vi "Pump_commands_Testcode.vi"() -> ()   [LabVIEW 2024]
uses:
  <vilib>/Instr/_visa.llb/VISA Find Search Mode.ctl
  ee3f6e9a-4254-40fb-8a6d-f40dbbb11eb6.vi
  <vilib>/regexp/Match Regular Expression.xnode
panel:
  out "element 2":u8
  out "element":u8
  out "read buffer":string
  out "Error":string
  out "Error present":bool
  out "Ready":bool
  out "Boolean array":bool[](array[boolean])
  out "Numeric 2":u8
  out "unsigned byte array":u8[](array[numeric])
  in  "Send":bool
  out "appended array":T1(array[ring])
  out "Responce array":string[](array[string])
  out "error out 2":errorcluster
  out "Numeric":i32
  out "Pump found":bool
  out "String":string
  in  "stop":bool
  in  "Enum":T2(ring)
  out "Array":string[](array[string])
  # "Hvis pumpen køre hurtigere end 17 laver den cavitations eller får væsken til at kåge"
  # "5"
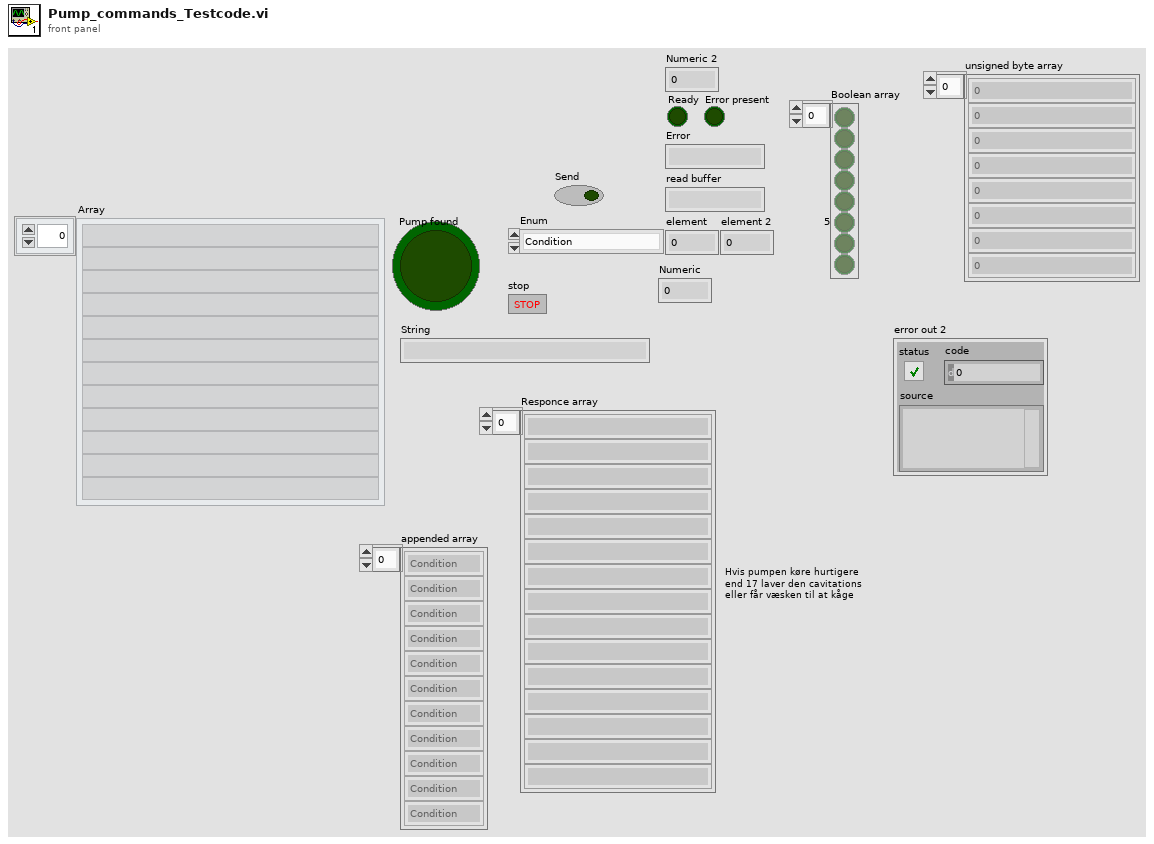
[diagram p1: front panel]
types:
  T1 = enum16{"Condition", "Pump out", "Pump in", "Initiate"}[]
  T2 = enum16{"Condition", "Pump out", "Pump in", "Initiate"}
  T3 = typedef "VISA Find Search Mode.ctl" = u32
  T4 = cluster{"VISA resource name":refnum<visa-resource-name>, "error out":errorcluster}
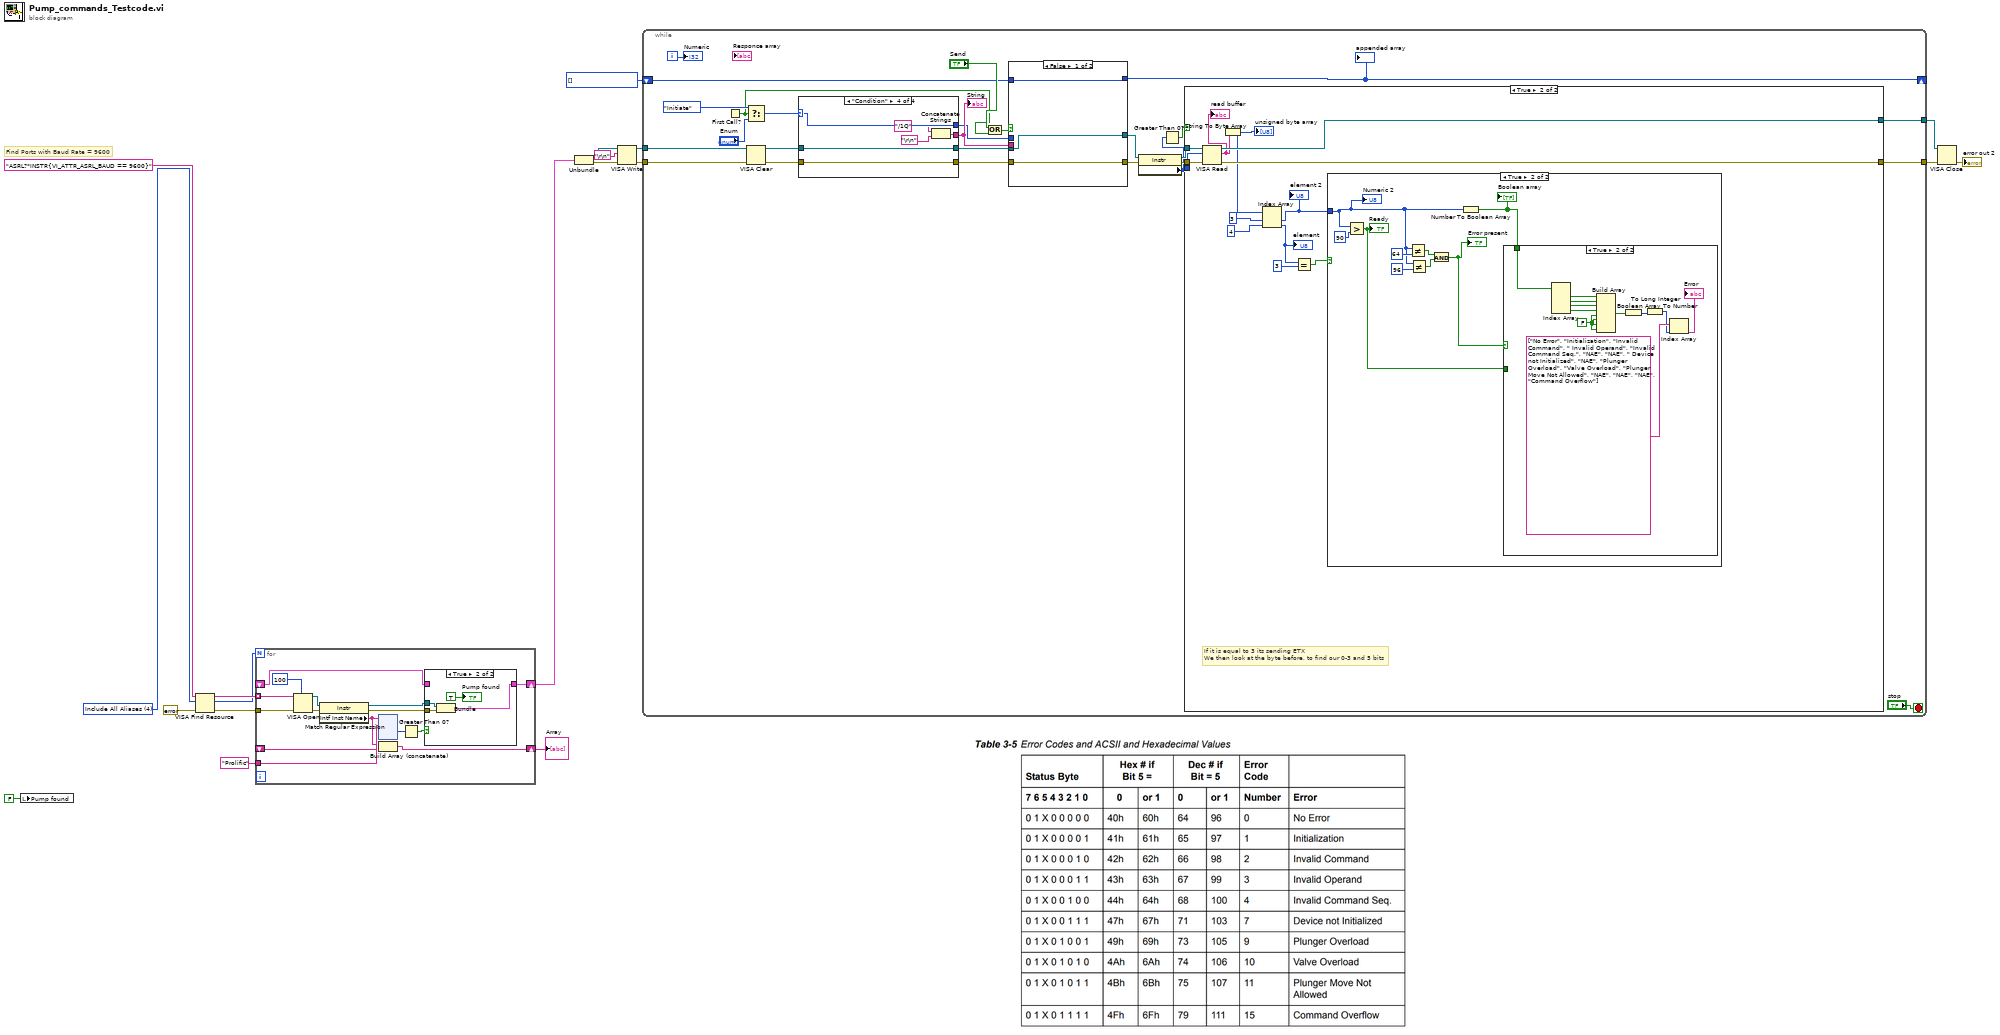
[diagram p0: block diagram]
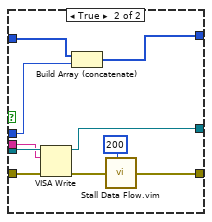
[diagram p5: hidden frame]
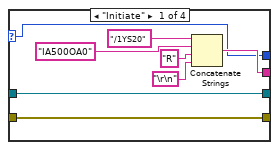
[diagram p6: hidden frame]
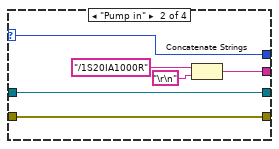
[diagram p7: hidden frame]
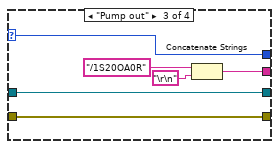
[diagram p8: hidden frame]
diagram:
  w1 = T1 [] items=["Condition", "Pump out", "Pump in", "Initiate"]
  w16 = T3 4 items=["Canonical Names Only"=0, "Aliases Only"=2, "Include Matching Aliases"=3, "Include All Aliases"=4] ("Search Mode")
  # "Find Ports with Baud Rate = 9600"
  n1 = local write "Pump found"(FALSE ("Pump found")) -> ()
  n2 = VISA Find Resource(8:errorcluster {"status"=FALSE, "code"=0, "source"=""} ("error in"), 10:w16, 11:"ASRL?*INSTR{VI_ATTR_ASRL_BAUD == 9600}" ("expression (\"?*\")")) -> (0:w18:errorcluster, 2:w11:u32, 3:w19:string[])
  n3 = for {
    N: w11 -> [_]
    tunnel: w19 -> [w34] mode=indexing
    tunnel: w18 -> [w31]
    shift-right: [w30] -> w14
    shift-left: _ -> [w29]
    tunnel: "Prolific" -> [w24]
    shift-right: [w21] -> w10
    shift-left: _ -> [w20]
    n4 = VISA Open(timeout (0)=u32 100 ("VISA Open timeout (0)"), error in (no error)=w31, VISA resource name=w34) -> (VISA resource name=w33:refnum<visa-resource-name>, error out=w32:errorcluster)  [unwired: 2 in]
    n5 = property class="Instr"(reference=w33, error in=w32) -> (reference out=w26:refnum<visa-resource-name>, error out=w25:errorcluster, "Intf Inst Name"=w22:string)
    n6 = xnode "Match Regular Expression"("input string"=w22, "regular expression"=w24) -> ("offset past match"=w28:i32)  [unwired: 4 in, 4 out]
    n7 = Build Array (concatenate)(w22, w20) -> (w21:string[])
    n8 = Greater Than 0?(x=w28) -> (x > 0?=w27:bool)
    n9 = case shown="True" w27 {
      tunnel: w26 -> [_ w156]
      tunnel: w25 -> [_ w155]
      tunnel: [w152 w154] -> w30
      tunnel: w29 -> [w152 _]
      frame False {
      }
      frame True {
        n10 = Bundle("VISA resource name"=w156, "error out"=w155) -> (w154:T4)  [unwired: 1 in]
        "Pump found" <- TRUE
      }
    }
  }
  "Array" <- w10
  n11 = Unbundle(w14) -> ("VISA resource name"=w8:refnum<visa-resource-name>, "error out"=w9:errorcluster)
  n12 = VISA Write(VISA resource name=w8, write buffer="\r\n", error in (no error)=w9) -> (VISA resource name out=w2:refnum<visa-resource-name>, error out=w3:errorcluster)  [unwired: 1 out]
  n13 = while {
    tunnel: [w177] -> w6
    tunnel: [w178] -> w5
    tunnel: w3 -> [w175]
    tunnel: w2 -> [w174]
    shift-right: [w159] -> _
    shift-left: w1 -> [w160]
    i -> [w181]
    stop <- "stop" stop-if-true
    n14 = First Call?() -> (First Call?: T/F=w163:bool)
    n15 = Select(t=T2."Initiate", s=w163, f="Enum") -> (s? t:f=w165:T2)
    n16 = VISA Clear(VISA resource name=w174, error in (no error)=w175) -> (VISA resource name out=w172:refnum<visa-resource-name>, error out=w173:errorcluster)
    n17 = case shown="\"Condition\"" w165 {
      selector: w165 -> [w231 w239 w245 w254]
      tunnel: [w238 w244 w250 w256] -> w170
      tunnel: w172 -> [w238 w244 w250 w256]
      tunnel: [w237 w243 w249 w255] -> w171
      tunnel: w173 -> [w237 w243 w249 w255]
      tunnel: [w233 w241 w246 w253] -> w168
      tunnel: [w231 w239 w245 w254] -> w161
      frame "Initiate" {
        n18 = Concatenate Strings("/1YS20", "IA500OA0" ("string"), "R" ("string"), "\r\n") -> (w233:string)
      }
      frame "Pump in" {
        n19 = Concatenate Strings("/1S20IA1000R", "\r\n") -> (w241:string)
      }
      frame "Pump out" {
        n20 = Concatenate Strings("/1S20OA0R", "\r\n") -> (w246:string)
      }
      frame "Condition" {
        n21 = Concatenate Strings("/1Q", "\r\n") -> (w253:string)
      }
    }
    "String" <- w168
    n22 = Or(x="Send", y=w163) -> (x .or. y?=w162:bool)
    n23 = case shown="False" w162 {
      tunnel: [w219 w222] -> w176
      tunnel: w171 -> [w219 w230]
      tunnel: w170 -> [w220 w229]
      tunnel: [w220 w228] -> w169
      tunnel: w168 -> [_ w227]
      tunnel: w161 -> [_ w224]
      tunnel: w160 -> [w218 w226]
      tunnel: [w218 w225] -> w159
      frame False {
      }
      frame True {
        n24 = VISA Write(VISA resource name=w229, write buffer=w227, error in (no error)=w230) -> (VISA resource name out=w228:refnum<visa-resource-name>, error out=w223:errorcluster)  [unwired: 1 out]
        n25 = Build Array (concatenate)(w226, w224) -> (w225:T1)
        n26 = call "Stall Data Flow.vim"("value in"=w223, "milliseconds to wait"=u32 200) -> ("value out"=w222:errorcluster)  [unwired: 1 out]
      }
    }
    "appended array" <- w159
    n27 = property class="Instr"(reference=w169, error in=w176) -> (reference out=w179:refnum<visa-resource-name>, error out=w180:errorcluster, "Serial Settings:Number of Bytes at Serial Port"=w158:u32)
    n28 = Greater Than 0?(x=w158) -> (x > 0?=w157:bool)
    n29 = case shown="True" w157 {
      tunnel: w180 -> [w183 w193]
      tunnel: w179 -> [w184 w194]
      tunnel: w158 -> [_ w197]
      tunnel: [w184 w196] -> w178
      tunnel: [w183 w195] -> w177
      frame False {
      }
      frame True {
        # "If it is equal to 3 its sending ETX\nWe then look at the byte before, to find our 0-3 and 5 bits"
        n30 = VISA Read(VISA resource name=w194, byte count=w197, error in (no error)=w193) -> (VISA resource name out=w196:refnum<visa-resource-name>, read buffer=w192:string, error out=w195:errorcluster)  [unwired: 1 out]
        "read buffer" <- w192
        n31 = String To Byte Array(string=w192) -> (unsigned byte array=w191:u8[])
        "unsigned byte array" <- w191
        n32 = Index Array(array=w191, index #1=3 ("index"), index #2=4 ("index")) -> (element #1=w185:u8, element #2=w187:u8)
        "element" <- w187
        "element 2" <- w185
        n33 = Equal?(x=w187, y=u8 3 ("x")) -> (x = y?=w186:bool)
        n34 = case shown="True" w186 {
          tunnel: w185 -> [_ w199]
          frame False {
          }
          frame True {
            n35 = Greater?(x=w199, y=u8 90) -> (0:w200:bool)
            "Ready" <- w200
            n36 = Not Equal?(x=w199, y=u8 64) -> (x != y?=w203:bool)
            n37 = Not Equal?(x=w199, y=u8 96) -> (x != y?=w202:bool)
            n38 = And(x=w203, y=w202) -> (x .and. y?=w201:bool)
            "Error present" <- w201
            n39 = Number To Boolean Array(number=w199) -> (Boolean array=w198:bool[])
            "Boolean array" <- w198
            n40 = case shown="True" w201 {
              tunnel: w200 -> [_ _]
              tunnel: w198 -> [_ w217]
              frame False {
              }
              frame True {
                w212 = FALSE
                n41 = Index Array(array=w217) -> (element #1=w216:bool, element #2=w215:bool, element #3=w214:bool, element #4=w213:bool)  [unwired: 4 in]
                n42 = Build Array(w216, w215, w214, w213, w212, w212, w212, w212) -> (w211:bool[])
                n43 = Boolean Array To Number(Boolean array=w211) -> (number=w209:u32)
                n44 = To Long Integer(number=w209) -> (32bit integer=w208:i32)
                n45 = Index Array(array=string[] ["No Error", "Initialization", "Invalid Command", " Invalid Operand", "Invalid Command Seq.", "NAE", "NAE", " Device not Initialized", "NAE", "Plunger Overload", "Valve Overload", "Plunger Move Not Allowed", "NAE", "NAE", "NAE", "Command Overflow"], index=w208) -> (element=→"Error":string)
              }
            }
            "Numeric 2" <- w199
          }
        }
      }
    }
    "Numeric" <- w181
  }
  n46 = VISA Close(VISA resource name=w5, error in (no error)=w6) -> (error out=→"error out 2":errorcluster)
